vi "test.vi"() -> ()   [LabVIEW 2011]
uses:
  GUI_Template/GUI_master/tcp_new_data_event.ctl
  GUI_Template/GUI_master/tcp new data cluster.ctl
panel:
  out "error IO 2":errorcluster
  in  "insert tag":bool=TRUE
  out "tcp data event":T1
  in  "GUIdevice 5":string="TS-dg535-2"
  in  "position::5":dbl=40.15 caption="Discharge delay A" format="%_4f"
  in  "delay.Channel_B::4":dbl=40.15 caption="Discharge delay B" format="%_4f"
  in  "GUIdevice 4":string="TS-dg535-1"
  in  "delay.Channel_A::4":dbl=40.15 caption="Discharge delay A" format="%_4f"
  in  "stop":bool
  # "TEST STAND GRAPHICAL USER INTERFACE"
  # "- SCREEN 1"
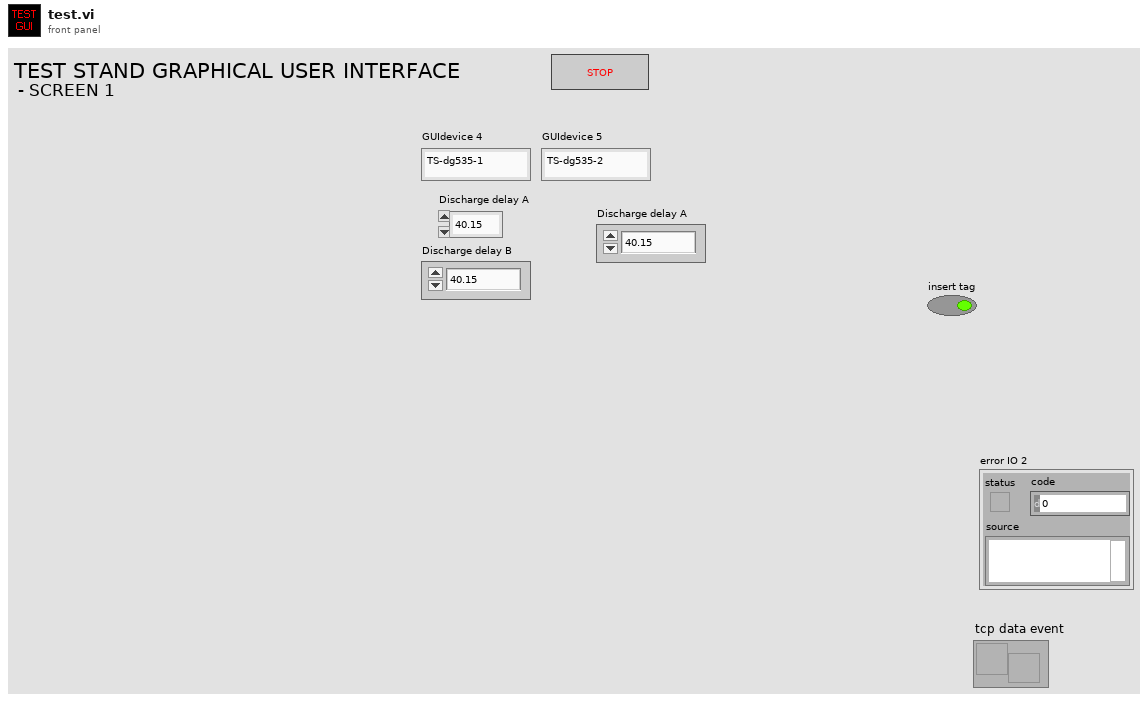
[diagram p1: front panel]
types:
  T1 = typedef "tcp_new_data_event.ctl" = refnum<user-event>
  T2 = typedef "tcp new data cluster.ctl" = cluster{"EventEnum":enum16{"new data", "connection status update"}, "Device name":string}
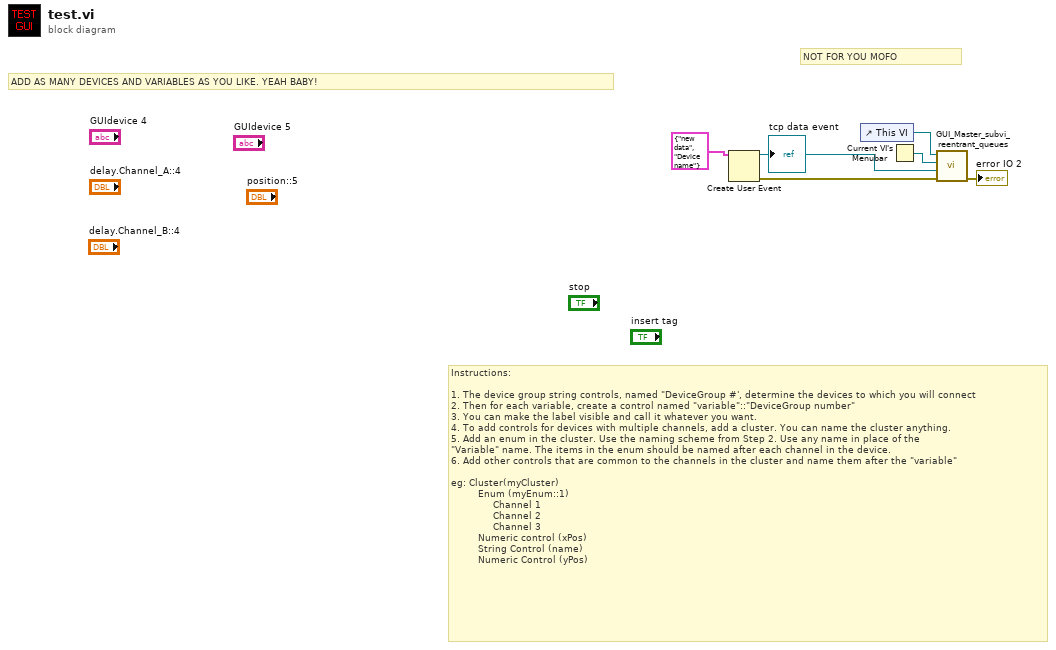
[diagram p0: block diagram]
diagram:
  # "Instructions:\n\n1. The device group string controls, named \"DeviceGroup #', determine the devices to which you will connect\n2. Then for each variable, create a control named \"variable\"::\"DeviceGroup number\"\n3. You can make the label visible and call it whatever you want.\n4. To add controls for devices with multiple channels, add a cluster. You can name the cluster anything.\n5. Add an enum in the cluster. Use the naming scheme from Step 2. Use any name in place of the \n\"Variable\" name. The items in the enum should be named after each channel in the device. \n6. Add other controls that are common to the channels in the cluster and name them after the \"variable\"\n\neg: Cluster(myCluster)\n         Enum (myEnum::1)\n              Channel 1 \n              Channel 2\n              Channel 3\n         Numeric control (xPos)\n         String Control (name)\n         Numeric Control (yPos)"
  # "ADD AS MANY DEVICES AND VARIABLES AS YOU LIKE. YEAH BABY!"
  # "NOT FOR YOU MOFO"
  n1 = Create User Event(user event datatype=T2 {"EventEnum"=enum."new data", "Device name"="Device name"} ("New Event")) -> (user event=w6:refnum<user-event>, error out=w5:errorcluster)  [unwired: 1 in]
  "tcp data event" <- w6
  n2 = control-ref of="This VI"() -> (w2:refnum<vi>)
  n3 = Current VI's Menubar() -> (w3:refnum<k9>)
  n4 = call "GUI_Master_subvi_reentrant_queues.vi"("error in (no error)"=w5, "tcp data event"=w6, "Caller menu reference"=w3, "Caller VI ref"=w2) -> ("error out"=→"error IO 2":errorcluster)  [unwired: 7 in]
